vi "CRYMR_Both_Margins.vi"(0 "Data":cluster{"Hz":dbl, "dB":dbl}[](array[cluster])=[{"Hz"=200.0, "dB"=4.5}, {"Hz"=1000.0, "dB"=5.0}, {"Hz"=5000.0, "dB"=6.0}] {"dB" format="%.1f"}, 1 "Upper Limit":cluster{"Hz":dbl, "y":dbl}[](array[cluster])=[{"Hz"=1000.0, "y"=3.0}] {"y" format="%.1f"}, 2 "Lower Limit":cluster{"Hz":dbl, "y":dbl}[](array[cluster])=[{"Hz"=1000.0, "y"=1.0}] {"y" format="%.1f"}) -> (3 "Upper Margin":dbl format="%.2f", 4 "Upper Margin X":dbl format="%.2f", 5 "Lower Margin":dbl format="%.2f", 6 "Lower Margin X":dbl format="%.2f")   [LabVIEW 2013]
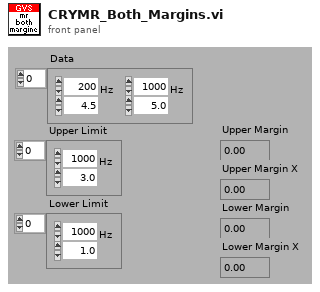
[diagram p1: front panel]
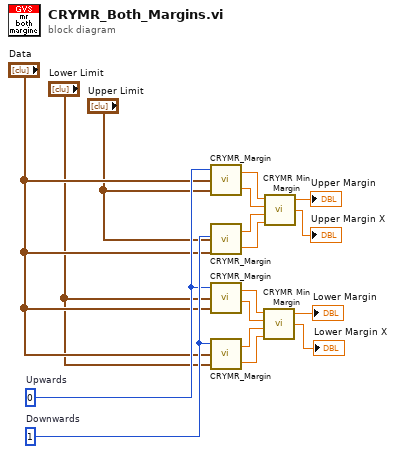
[diagram p0: block diagram]
diagram:
  w17 = 1  # Downwards
  w16 = 0  # Upwards
  n1 = call "CRYMR_Margin.vi"("To"="Upper Limit", "From"="Data", "Direction"=w16) -> ("X"=w8:dbl, "Margin"=w13:dbl)
  n2 = call "CRYMR_Margin.vi"("To"="Data", "From"="Upper Limit", "Direction"=w17) -> ("X"=w6:dbl, "Margin"=w7:dbl)
  n3 = call "CRYMR_Margin.vi"("To"="Data", "From"="Lower Limit", "Direction"=w16) -> ("X"=w9:dbl, "Margin"=w12:dbl)
  n4 = call "CRYMR_Margin.vi"("To"="Lower Limit", "From"="Data", "Direction"=w17) -> ("X"=w5:dbl, "Margin"=w11:dbl)
  n5 = call "CRYMR Min Margin.vi"("Lower X"=w5, "Lower Margin"=w11, "Upper X"=w9, "Upper Margin"=w12) -> ("X"=→"Lower Margin X":dbl, "Min Margin"=→"Lower Margin":dbl)  [unwired: 1 out]
  n6 = call "CRYMR Min Margin.vi"("Lower X"=w6, "Lower Margin"=w7, "Upper X"=w8, "Upper Margin"=w13) -> ("X"=→"Upper Margin X":dbl, "Min Margin"=→"Upper Margin":dbl)  [unwired: 1 out]
